vi "niWLAN - 80211Measure.vi"(0 "niwlan analysis session":T1, 5 "instrument handle":refnum<k15>, 9 "timeout (10 sec)":dbl=10.0, 11 "error in":errorcluster) -> (4 "niwlan analysis session out":T1, 6 "instrument handle out":refnum<k15>, 15 "error out":errorcluster {"code" format="%.0x"})   [LabVIEW 2012]
uses:
  <vilib>/RF Toolkits/WLAN/analysis/controls/wlanv1 Analysis Refnum.ctl
  <vilib>/RF Toolkits/WLAN/analysis/subVIs/Measure/niWLANA RFSA Single Channel Measure.vi
  <vilib>/RF Toolkits/WLAN/analysis/subVIs/Measure/niWLANA RFSA Multiple Channel Measure.vi
  <resource>/objmgr/niWLANAnalysis.rc
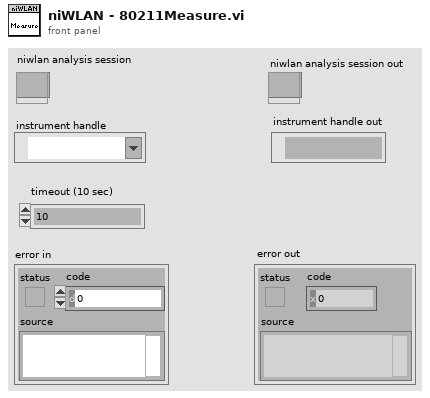
[diagram p1: front panel]
types:
  T1 = typedef "wlanv1 Analysis Refnum.ctl" = refnum<k20>
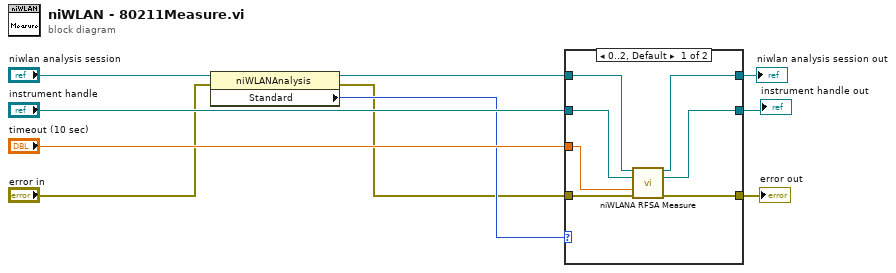
[diagram p0: block diagram]
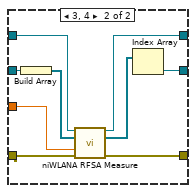
[diagram p2: hidden frame]
diagram:
  n1 = property class="niWLANAnalysis"(reference="niwlan analysis session", error in="error in") -> (reference out=w4:T1, error out=w1:errorcluster, "Standard"=w3:i32)
  n2 = case shown="0..2, Default" w3 {
    tunnel: [w17 w26] -> w6
    tunnel: w1 -> [w16 w25]
    tunnel: w4 -> [w15 w24]
    tunnel: [w12 w23] -> w10
    tunnel: "instrument handle" -> [w13 w22]
    tunnel: [w11 w19] -> w8
    tunnel: "timeout (10 sec)" -> [w14 w18]
    frame 0..2, Default {
      n3 = call-poly <vilib>:"niWLANA RFSA Measure.vi"("niwlan analysis session"=w15, "instrument handle"=w13, "timeout (10 sec)"=w14, "error in"=w16) -> ("niwlan analysis session out"=w12:T1, "instrument handle out"=w11:refnum<k15>, "error out"=w17:errorcluster)  [unwired: 9 out]
    }
    frame 3, 4 {
      n4 = Build Array(w22) -> (w21:refnum<k15>[])
      n5 = call-poly <vilib>:"niWLANA RFSA Measure.vi"("niwlan analysis session"=w24, "instrument handles"=w21, "timeout (10 sec)"=w18, "error in"=w25) -> ("niwlan analysis session out"=w23:T1, "instrument handles out"=w20:refnum<k15>[], "error out"=w26:errorcluster)  [unwired: 9 out]
      n6 = Index Array(array=w20) -> (element=w19:refnum<k15>)  [unwired: 1 in]
    }
  }
  "niwlan analysis session out" <- w10
  "instrument handle out" <- w8
  "error out" <- w6
